vi "Init.vi"(8 "error in (no error)":errorcluster, 9 "Type":u16(ring) items=["人脑", "电脑"], 10 "Name":u16(ring) items=["玩家1", "玩家2"], 11 "Player in":refnum<class "Player.lvclass">) -> (0 "error out":errorcluster, 3 "Player out":refnum<class "Player.lvclass">)   [LabVIEW 2009, in "Player.lvclass"]
doc: "The Initialize the Player Class."
uses:
  Player.lvclass
  Player.lvclass/Player.ctl
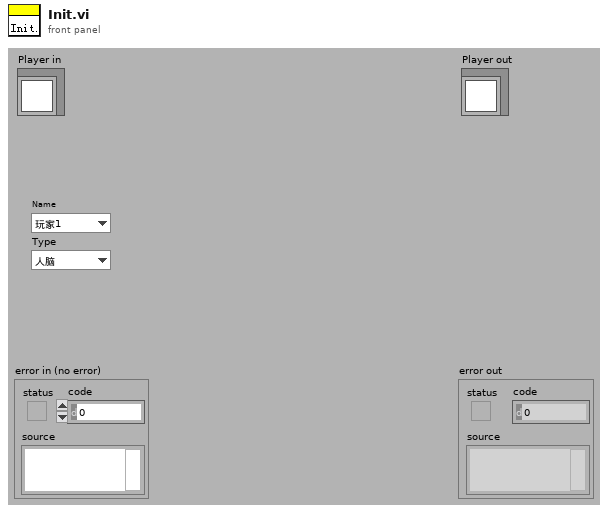
[diagram p1: front panel]
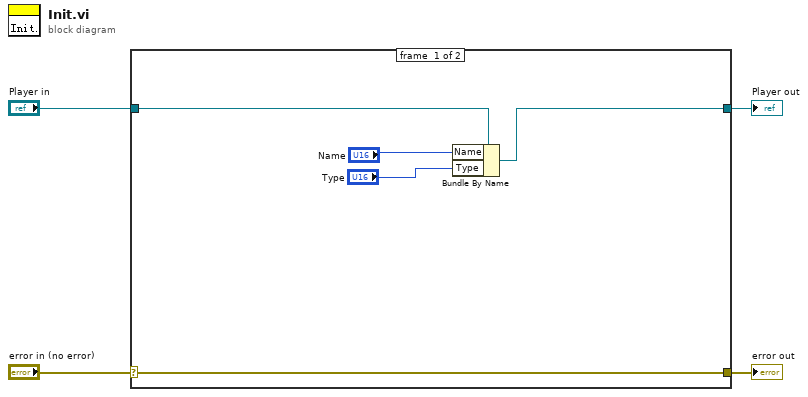
[diagram p0: block diagram]
diagram:
  n1 = case shown="No Error" "error in (no error)" {
    selector: "error in (no error)" -> [w9 w11]
    tunnel: [w9 w11] -> w3
    tunnel: [w7 w10] -> w1
    tunnel: "Player in" -> [w8 w10]
    frame #0 {
      n2 = Bundle By Name(cluster=w8, "Name"="Name", "Type"="Type") -> (w7:refnum<class "Player.lvclass">)
    }
    frame #1 {
    }
  }
  "error out" <- w3
  "Player out" <- w1
